vi "RedOrGreen.vi"(1 "success":bool) -> (0 "color":string)   [LabVIEW 2018]
doc: "Changes the color to red or green depending on the state (success=green)"
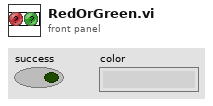
[diagram p1: front panel]
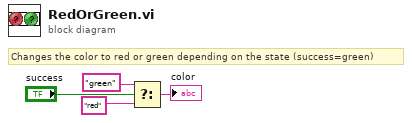
[diagram p0: block diagram]
diagram:
  # "Changes the color to red or green depending on the state (success=green)"
  n1 = Select(t="green" ("format string"), s="success", f="red" ("format string")) -> (s? t:f=→"color":string)
